vi "Dereference NULL-Terminated String.vi"(8 "error in (no error)":errorcluster, 11 "char*":u64) -> (0 "error out":errorcluster, 2 "string":string)   [LabVIEW 2017, in "libssh2.lvlib"]
uses:
  libssh2.lvlib
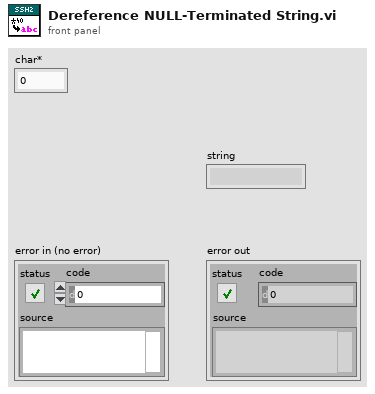
[diagram p1: front panel]
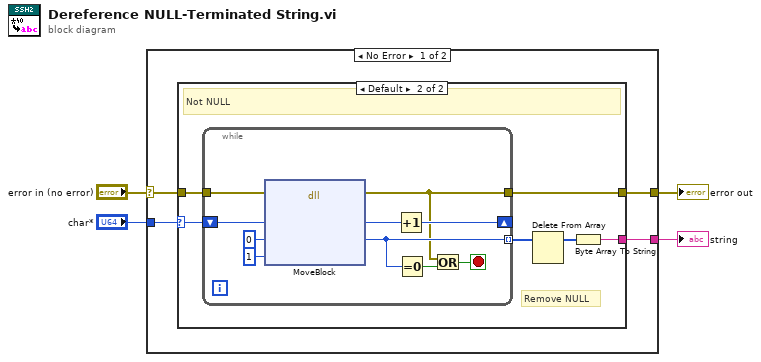
[diagram p0: block diagram]
diagram:
  n1 = case shown="No Error" "error in (no error)" {
    selector: "error in (no error)" -> [w6 w26]
    tunnel: [w8 _] -> w4
    tunnel: "char*" -> [w7 _]
    tunnel: [w5 w26] -> w1
    frame No Error {
      n2 = case shown="Default" w7 {
        selector: w7 -> [_ w13]
        tunnel: [_ w14] -> w8
        tunnel: w6 -> [w9 w12]
        tunnel: [w9 w11] -> w5
        frame 0 {
          # "NULL"
        }
        frame Default {
          # "Remove NULL"
          # "Not NULL"
          n3 = while {
            tunnel: [w18] -> w15 mode=indexing
            shift-right: [w21] -> _
            shift-left: w13 -> [w25]
            tunnel: w12 -> [w20]
            tunnel: [w16] -> w11
            stop <- w19 stop-if-true
            n4 = dll-call lib="LabVIEW" fn="MoveBlock"(error in=w20, "ps"=w25, "pd"=u8 0, "size"=u64 1) -> (error out=w16:errorcluster, "ps"=w22:u64, "pd"=w18:u8)  [unwired: 4 in, 1 out]
            n5 = Increment(x=w22) -> (x+1=w21:u64)
            n6 = Equal To 0?(x=w18) -> (x = 0?=w17:bool)
            n7 = Or(x=w16, y=w17) -> (x .or. y?=w19:bool)
          }
          n8 = Delete From Array(array=w15) -> (array with subset deleted=w10:u8[])  [unwired: 2 in, 1 out]
          n9 = Byte Array To String(unsigned byte array=w10) -> (string=w14:string)
        }
      }
    }
    frame Error {
    }
  }
  "string" <- w4
  "error out" <- w1
